vi "Screen_Setup.vi"() -> ()   [LabVIEW 2010]
uses:
  Locked Config.ctl
  030 - EVENTS/EnumFgvEventCommand.ctl
  090 - ERRORS/Ctrls/enumLogAndView.ctl
  <vilib>/Utility/miscctls.llb/LVComboBoxStrsAndValuesArrayTypeDef.ctl
  050 - CONFIG/00 - ApplicationConfig/Ctrls/EnumFgvConfigCommand.ctl
  080 - TOOLS/Traduction/Dictionnary/EnumCommandDictionnaire.ctl
  030 - EVENTS/03 - ToMessageHandlerProcess/enumMessageCriticity.ctl
  030 - EVENTS/03 - ToMessageHandlerProcess/ToMessageHandlerEvent.ctl
  enumScreen.ctl
panel:
  in  "Locked ?":T1
  in  "Répertoire des données":path
  in  "Langue":string(combo)
  in  "Nombre MAX de message par fichier":u16
  in  "Nombre max de fichiers LOG":u16
  in  "Cfg":string
  in  "Bouton menu principal":bool
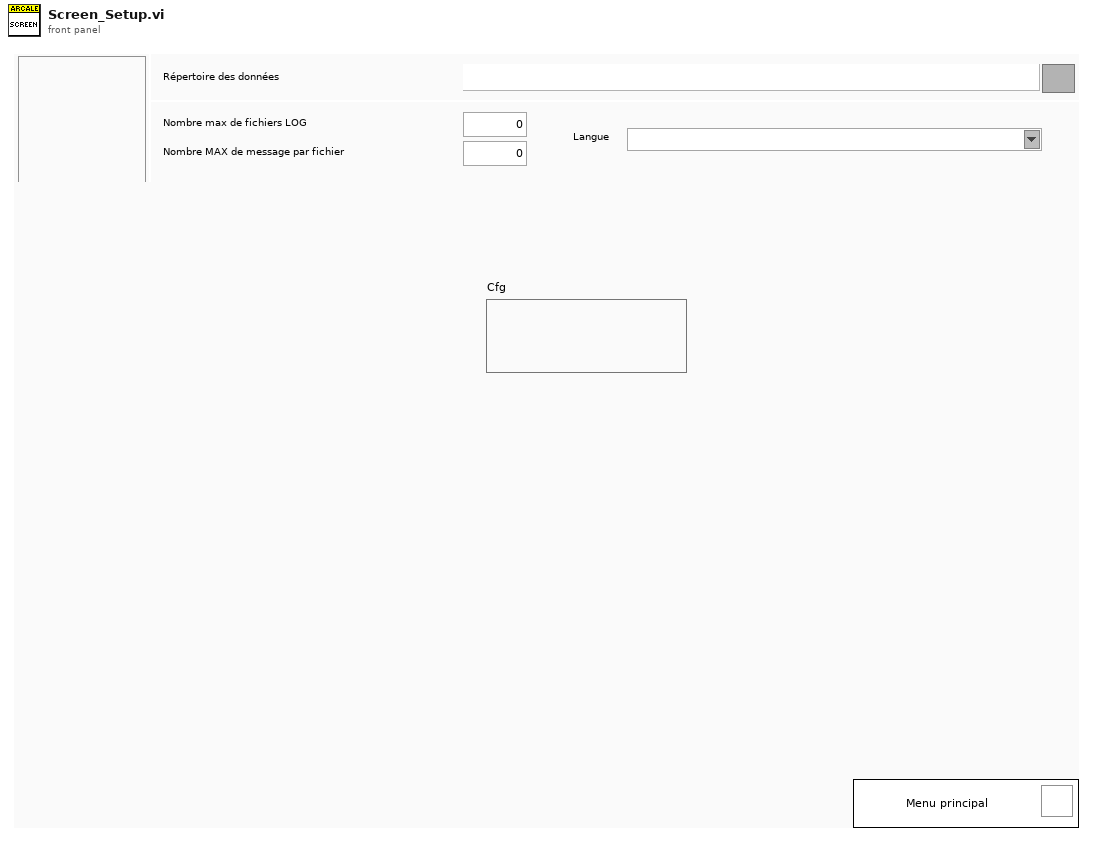
[diagram p1: front panel]
types:
  T1 = typedef "Locked Config.ctl" = bool
  T2 = typedef "enumLogAndView.ctl" = enum16{"Log only", "Log and view"}
  T3 = typedef "EnumFgvEventCommand.ctl" = enum16{"Setup", "Cleanup", "Get"}
  T4 = typedef "LVComboBoxStrsAndValuesArrayTypeDef.ctl" = cluster{"String":string, "Value":string}[]
  T5 = typedef "EnumFgvConfigCommand.ctl" = enum16{"Load", "Get", "Set", "Save To Disk"}
  T6 = typedef "ApplicationConfig.ctl" = cluster{"Data Path":path, "MessageHandlerConfig":T7, "Simulation":bool, "Dictionnary":string}
  T7 = typedef "MessageHandlerConfig.ctl" = cluster{"Max log files":u32, "Max messages per file":u32}
  T8 = typedef "BenchConfig.ctl" = cluster{"Cfg":string}
  T9 = enum8{"Enabled", "Disabled", "Disabled and Grayed Out"}
  T10 = typedef "EnumCommandDictionnaire.ctl" = enum16{"Load", "Translate", "Save", "GetDico", "Set : A traduire = Vrai", "Set : A Traduire = Faux", "SetDico"}
  T11 = typedef "enumMessageCriticity.ctl" = enum16{"No error", "Info", "Warning", "Error", "Fatal error"}
  T12 = typedef "ToMessageHandlerEvent.ctl" = cluster{"date / time":timestamp, "Criticity":T11, "Emitter":string, "Message":string}
  T13 = typedef "enumScreen.ctl" = enum16{"Test screen", "Ecran principal", "LOG", "Setup", "Popup : About", "Popup : View last message", "Popup : WebBrowser help", "Traduction"}
  T14 = typedef "ToScreensCommand.ctl" = enum16{"Stop screen", "Stop all screens"}
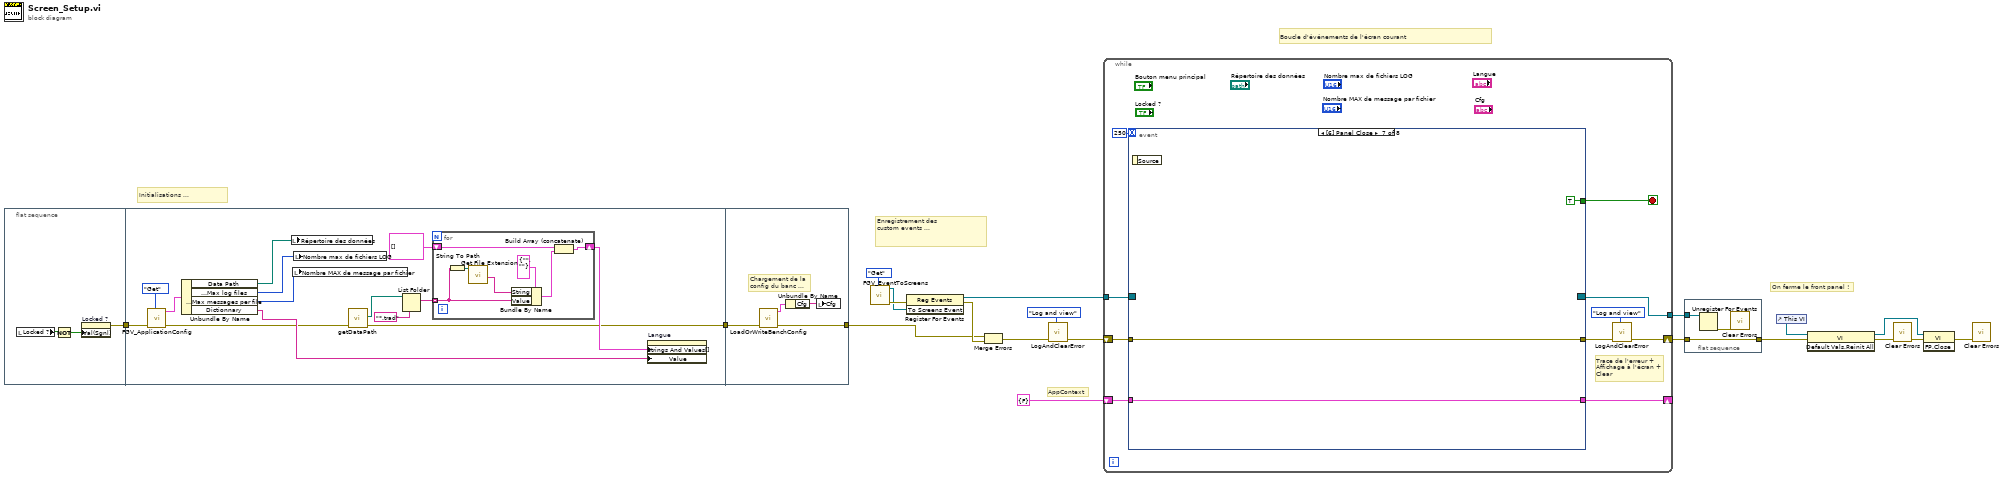
[diagram p0: block diagram]
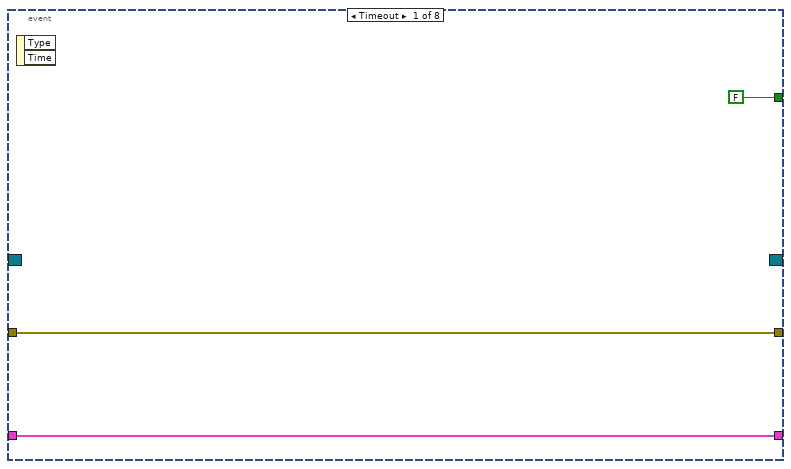
[diagram p2: hidden frame]
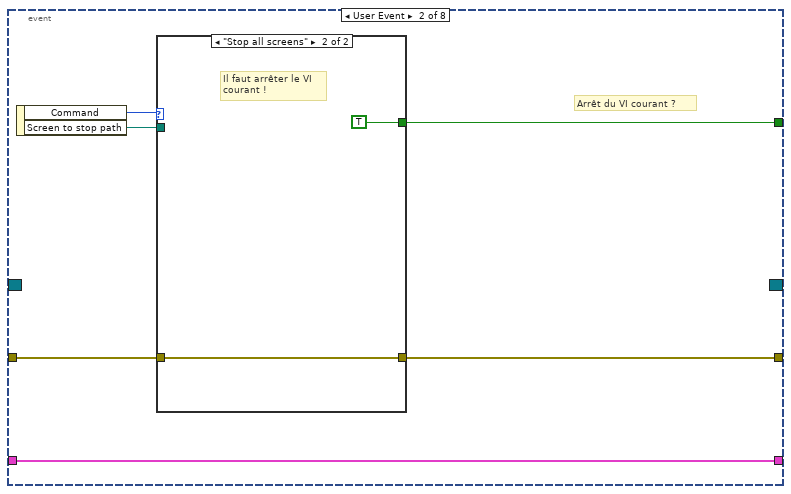
[diagram p3: hidden frame]
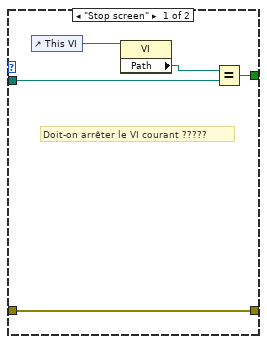
[diagram p4: hidden frame]
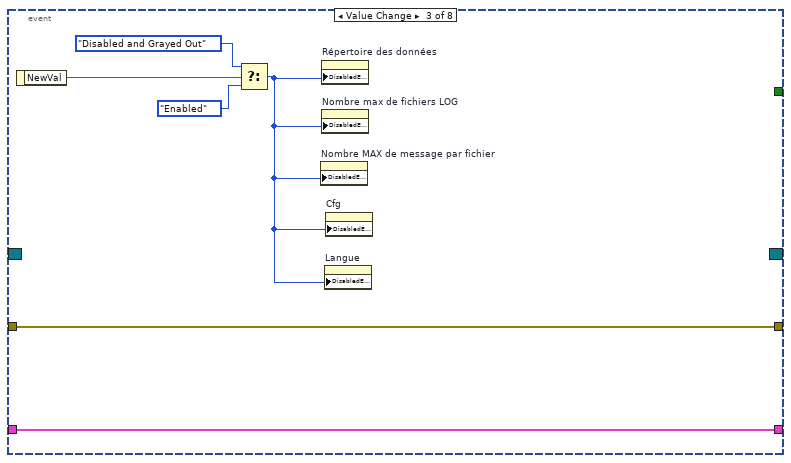
[diagram p5: hidden frame]
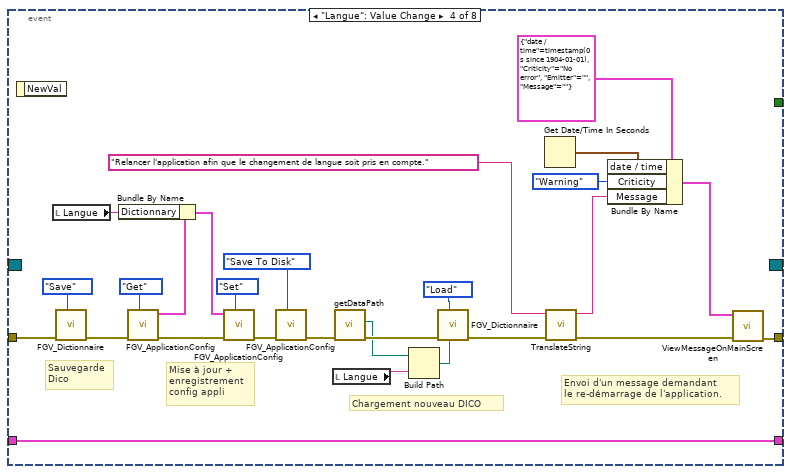
[diagram p6: hidden frame]
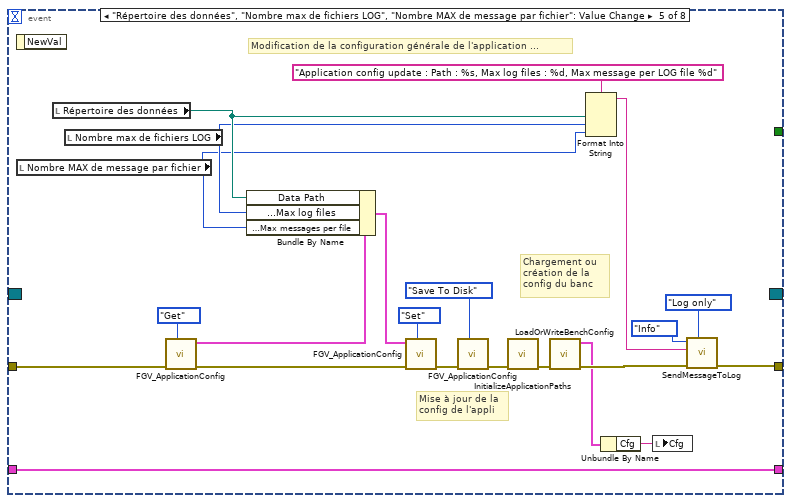
[diagram p7: hidden frame]
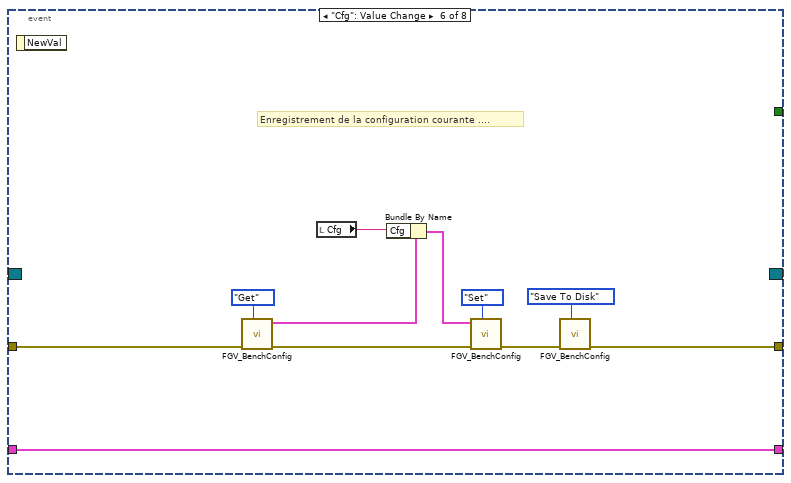
[diagram p8: hidden frame]
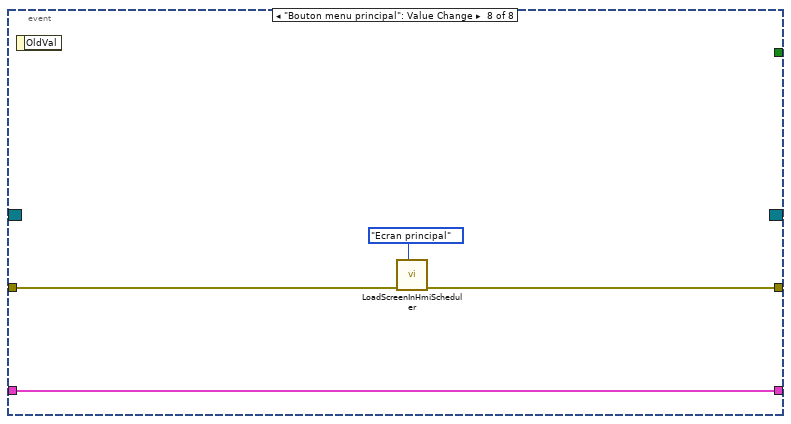
[diagram p9: hidden frame]
diagram:
  # "AppContext"
  # "Enregistrement des\ncustom events ..."
  # "Initialisations ..."
  # "On ferme le front panel !"
  # "Boucle d'événements de l'écran courant"
  n1 = flat-sequence {
    tunnel: [w23] -> w10
    tunnel: w10 -> [w36]
    tunnel: [w25] -> w9
    tunnel: [w47] -> w11
    tunnel: w9 -> [w48]
    frame #0 {
      n2 = local read "Locked ?"() -> (w21:T1)
      n3 = Not(x=w21) -> (.not. x?=w22:T1)
      n4 = property on="Locked ?" class="Bool (strict)"("Val(Sgnl)"=w22) -> (error out=w23:errorcluster)  [unwired: 2 in, 1 out]
    }
    frame #1 {
      n5 = call "FGV_ApplicationConfig.vi"("Command"=EnumFgvConfigCommand."Get", "error in (no error)"=w36) -> ("error out"=w26:errorcluster, "ApplicationConfigOut"=w35:T6)  [unwired: 8 in]
      n6 = Unbundle By Name(w35) -> ("Data Path"=w32:path, "MessageHandlerConfig.Max log files"=w34:u32, "MessageHandlerConfig.Max messages per file"=w33:u32, "Dictionnary"=w30:string)
      n7 = local write "Répertoire des données"(w32) -> ()
      n8 = local write "Nombre MAX de message par fichier"(w33) -> ()
      n9 = local write "Nombre max de fichiers LOG"(w34) -> ()
      n10 = call "getDataPath.vi"("error in (no error)"=w26) -> ("error out"=w25:errorcluster, "DataPath"=w24:path)  [unwired: 9 in]
      n11 = List Folder(path=w24, pattern="*.trad") -> (filenames=w29:string[])  [unwired: 2 in, 3 out]
      n12 = for {
        tunnel: w29 -> [w40] mode=indexing
        shift-right: [w43] -> w27
        shift-left: T4 [] ("Strings And Values []") -> [w44]
        n13 = String To Path(string=w40) -> (path=w39:path)
        n14 = call <vilib>:"Get File Extension.vi"("file"=w39) -> ("filename without extension"=w38:string)  [unwired: 7 in, 3 out]
        n15 = Bundle By Name(cluster=cluster{"String":string, "Value":string} {"String"="", "Value"=""}, "String"=w38, "Value"=w40) -> (w41:cluster{"String":string, "Value":string})
        n16 = Build Array (concatenate)(w44, w41) -> (w43:T4)
      }
      n17 = property on="Langue" class="CmbBox"("Strings And Values[]"=w27, "Value"=w30) -> ()  [unwired: 2 in, 2 out]
    }
    frame #2 {
      # "Chargement de la \nconfig du banc ..."
      n18 = call "LoadOrWriteBenchConfig.vi"("error in (no error)"=w48) -> ("error out"=w47:errorcluster, "BenchConfig"=w46:T8)  [unwired: 9 in]
      n19 = Unbundle By Name(w46) -> ("Cfg"=w45:string)
      n20 = local write "Cfg"(w45) -> ()
    }
  }
  n21 = call "FGV_EventToScreens.vi"("Command"=EnumFgvEventCommand."Get") -> ("error out"=w20:errorcluster, "To Screens Event"=w19:refnum<user-event>)  [unwired: 9 in]
  n22 = register-events(error in=w20, w19) -> (reference out=w18:refnum<event-registration>, error out=w13:errorcluster)  [unwired: 1 in]
  n23 = Merge Errors(w11, w13) -> (w7:errorcluster)
  n24 = call "LogAndClearError.vi"("Log and view ?"=enumLogAndView."Log and view", "error in (no error)"=w7) -> ("error out"=w6:errorcluster)  [unwired: 9 in]
  n25 = while {
    tunnel: w18 -> [w58]
    shift-right: [w52] -> w16
    shift-left: w6 -> [w57]
    tunnel: [w56] -> w17
    shift-right: [w53] -> _
    shift-left: cluster{"Boolean":bool} {"Boolean"=FALSE} ("Cluster") -> [w54]
    stop <- w55 stop-if-true
    # "Trace de l'erreur +\nAffichage à l'écran +\nClear"
    n26 = event shown="[6] Panel Close" {
      selector: w58 -> [_ _ _ _ _ _ _ _]
      dyn-events: [_ _ _ _ _ _ _ _] -> w56
      timeout: 250 -> [_ _ _ _ _ _ _ _]
      tunnel: w57 -> [w61 w66 w77 w90 w127 w139 w142 w147]
      tunnel: [w61 w65 w77 w97 w123 w133 w142 w145] -> w51
      tunnel: [FALSE w63 _ _ _ _ TRUE _] -> w55
      tunnel: w54 -> [w59 w62 w76 w107 w122 w138 w141 w144]
      tunnel: [w59 w62 w76 w107 w122 w138 w141 w144] -> w53
      event Timeout {
        n27 = event-data() -> ()  [unwired: 1 in, 2 out]
      }
      event User Event {
        # "Arrêt du VI courant ?"
        n28 = event-data() -> ("Command"=w67:T14, "Screen to stop path"=w64:path)  [unwired: 1 in]
        n29 = case shown="\"Stop all screens\"" w67 {
          tunnel: w66 -> [w72 w73]
          tunnel: [w72 w73] -> w65
          tunnel: w64 -> [w69 _]
          tunnel: [w68 TRUE] -> w63
          frame "Stop screen" {
            # "Doit-on arrêter le VI courant ?????"
            n30 = control-ref of="This VI"() -> (w71:refnum<vi>)
            n31 = property class="VI"(reference=w71) -> ("Path"=w70:path)  [unwired: 1 in, 2 out]
            n32 = Equal?(x=w70, y=w69) -> (x = y?=w68:bool)
          }
          frame "Stop all screens" {
            # "Il faut arrêter le VI\ncourant !"
          }
        }
      }
      event Value Change {
        n33 = event-data() -> ("NewVal"=w80:T1)  [unwired: 1 in]
        n34 = Select(t=T9."Disabled and Grayed Out" ("Disabled"), s=w80, f=T9."Enabled" ("Disabled")) -> (s? t:f=w75:T9)
        n35 = property on="Nombre MAX de message par fichier" class="DigNum (strict)"("DisabledEnum"=w75) -> ()  [unwired: 2 in, 2 out]
        n36 = property on="Répertoire des données" class="Path"("DisabledEnum"=w75) -> ()  [unwired: 2 in, 2 out]
        n37 = property on="Nombre max de fichiers LOG" class="DigNum (strict)"("DisabledEnum"=w75) -> ()  [unwired: 2 in, 2 out]
        n38 = property on="Langue" class="CmbBox"("DisabledEnum"=w75) -> ()  [unwired: 2 in, 2 out]
        n39 = property on="Cfg" class="Str"("DisabledEnum"=w75) -> ()  [unwired: 2 in, 2 out]
      }
      event "Langue": Value Change {
        # "Envoi d'un message demandant\nle re-démarrage de l'application."
        # "Chargement nouveau DICO"
        # "Mise à jour +\nenregistrement\nconfig appli"
        # "Sauvegarde\nDico"
        n40 = event-data() -> ()  [unwired: 1 in, 1 out]
        n41 = local read "Langue"() -> (w99:string)
        n42 = call "FGV_Dictionnaire.vi"("Command"=EnumCommandDictionnaire."Save", "error in (no error)"=w90) -> ("error out"=w89:errorcluster)  [unwired: 7 in, 2 out]
        n43 = call "FGV_ApplicationConfig.vi"("Command"=EnumFgvConfigCommand."Get", "error in (no error)"=w89) -> ("error out"=w104:errorcluster, "ApplicationConfigOut"=w101:T6)  [unwired: 8 in]
        n44 = Bundle By Name(cluster=w101, "Dictionnary"=w99) -> (w100:T6)
        n45 = call "FGV_ApplicationConfig.vi"("Command"=EnumFgvConfigCommand."Set", "error in (no error)"=w104, "ApplicationConfigIn"=w100) -> ("error out"=w102:errorcluster)  [unwired: 7 in, 1 out]
        n46 = call "FGV_ApplicationConfig.vi"("Command"=EnumFgvConfigCommand."Save To Disk", "error in (no error)"=w102) -> ("error out"=w85:errorcluster)  [unwired: 8 in, 1 out]
        n47 = local read "Langue"() -> (w82:string)
        n48 = call "getDataPath.vi"("error in (no error)"=w85) -> ("error out"=w84:errorcluster, "DataPath"=w83:path)  [unwired: 9 in]
        n49 = Build Path(base path=w83, name or relative path=w82) -> (appended path=w81:path)
        n50 = call "FGV_Dictionnaire.vi"("FichierDictionnaire"=w81, "Command"=EnumCommandDictionnaire."Load", "error in (no error)"=w84) -> ("error out"=w86:errorcluster)  [unwired: 6 in, 2 out]
        n51 = Get Date/Time In Seconds() -> (seconds since 1Jan1904=w94:timestamp)
        n52 = call "TranslateString.vi"("error in (no error)"=w86, "String"="Relancer l'application afin que le changement de langue soit pris en compte.") -> ("error out"=w98:errorcluster, "Translated String"=w92:string)  [unwired: 8 in]
        n53 = Bundle By Name(cluster=T12 {"date / time"=timestamp(0 s since 1904-01-01), "Criticity"=enum."No error", "Emitter"="", "Message"=""} ("Message"), "date / time"=w94, "Criticity"=enumMessageCriticity."Warning", "Message"=w92) -> (w95:T12)
        n54 = call "ViewMessageOnMainScreen.vi"("error in (no error)"=w98, "Message"=w95) -> ("error out"=w97:errorcluster)  [unwired: 9 in]
      }
      event "Répertoire des données", "Nombre max de fichiers LOG", "Nombre MAX de message par fichier": Value Change {
        # "Chargement ou\ncréation de la \nconfig du banc"
        # "Mise à jour de la\nconfig de l'appli"
        # "Modification de la configuration générale de l'application ..."
        n55 = event-data() -> ()  [unwired: 1 in, 1 out]
        n56 = local read "Nombre MAX de message par fichier"() -> (w115:u16)
        n57 = local read "Répertoire des données"() -> (w117:path)
        n58 = local read "Nombre max de fichiers LOG"() -> (w116:u16)
        n59 = call "FGV_ApplicationConfig.vi"("Command"=EnumFgvConfigCommand."Get", "error in (no error)"=w127) -> ("error out"=w126:errorcluster, "ApplicationConfigOut"=w125:T6)  [unwired: 8 in]
        n60 = Bundle By Name(cluster=w125, "Data Path"=w117, "MessageHandlerConfig.Max log files"=w116, "MessageHandlerConfig.Max messages per file"=w115) -> (w124:T6)
        n61 = call "FGV_ApplicationConfig.vi"("Command"=EnumFgvConfigCommand."Set", "error in (no error)"=w126, "ApplicationConfigIn"=w124) -> ("error out"=w111:errorcluster)  [unwired: 7 in, 1 out]
        n62 = call "FGV_ApplicationConfig.vi"("Command"=EnumFgvConfigCommand."Save To Disk", "error in (no error)"=w111) -> ("error out"=w110:errorcluster)  [unwired: 8 in, 1 out]
        n63 = call "InitializeApplicationPaths.vi"("error in (no error)"=w110) -> ("error out"=w114:errorcluster)  [unwired: 10 in]
        n64 = call "LoadOrWriteBenchConfig.vi"("error in (no error)"=w114) -> ("error out"=w113:errorcluster, "BenchConfig"=w108:T8)  [unwired: 9 in]
        n65 = Format Into String(format string="Application config update : Path : %s, Max log files : %d, Max message per LOG file %d", w117, w116, w115) -> (resulting string=w118:string)  [unwired: 2 in, 1 out]
        n66 = Unbundle By Name(w108) -> ("Cfg"=w109:string)
        n67 = local write "Cfg"(w109) -> ()
        n68 = call "SendMessageToLog.vi"("Log and view ?"=enumLogAndView."Log only", "error in (no error)"=w113, "Message"=w118, "Criticity"=enumMessageCriticity."Info") -> ("error out"=w123:errorcluster)  [unwired: 7 in]
      }
      event "Cfg": Value Change {
        # "Enregistrement de la configuration courante ...."
        n69 = event-data() -> ()  [unwired: 1 in, 1 out]
        n70 = call "FGV_BenchConfig.vi"("Command"=EnumFgvConfigCommand."Get", "error in (no error)"=w139) -> ("error out"=w136:errorcluster, "BenchConfigOut"=w132:T8)  [unwired: 8 in]
        n71 = local read "Cfg"() -> (w130:string)
        n72 = Bundle By Name(cluster=w132, "Cfg"=w130) -> (w131:T8)
        n73 = call "FGV_BenchConfig.vi"("Command"=EnumFgvConfigCommand."Set", "error in (no error)"=w136, "BenchConfigIn"=w131) -> ("error out"=w134:errorcluster)  [unwired: 7 in, 1 out]
        n74 = call "FGV_BenchConfig.vi"("Command"=EnumFgvConfigCommand."Save To Disk", "error in (no error)"=w134) -> ("error out"=w133:errorcluster)  [unwired: 8 in, 1 out]
      }
      event Panel Close {
        n75 = event-data() -> ()  [unwired: 1 in, 1 out]
      }
      event "Bouton menu principal": Value Change {
        n76 = event-data() -> ()  [unwired: 1 in, 1 out]
        n77 = call "LoadScreenInHmiScheduler.vi"("Enum Screen"=enumScreen."Ecran principal", "error in (no error)"=w147) -> ("error out"=w145:errorcluster)  [unwired: 9 in]
      }
    }
    n78 = call "LogAndClearError.vi"("Log and view ?"=enumLogAndView."Log and view", "error in (no error)"=w51) -> ("error out"=w52:errorcluster)  [unwired: 9 in]
  }
  n79 = flat-sequence {
    tunnel: w17 -> [w150]
    tunnel: w16 -> [w148]
    tunnel: [w148] -> w3
    frame #0 {
      n80 = Unregister For Events(event registration refnum=w150) -> (error out=w149:errorcluster)  [unwired: 1 in]
      n81 = call <vilib>:"Clear Errors.vi"("error in (no error)"=w149) -> ()  [unwired: 6 in, 1 out]
    }
  }
  n82 = control-ref of="This VI"() -> (w2:refnum<vi>)
  n83 = invoke class="VI" method="Default Vals.Reinit All"(reference=w2, error in=w3) -> (reference out=w1:refnum<vi>, error out=w5:errorcluster)  [unwired: 1 in, 1 out]
  n84 = call <vilib>:"Clear Errors.vi"("error in (no error)"=w5) -> ("error out"=w4:errorcluster)  [unwired: 6 in]
  n85 = invoke class="VI" method="FP.Close"(reference=w1, error in=w4) -> (error out=w15:errorcluster)  [unwired: 1 in, 2 out]
  n86 = call <vilib>:"Clear Errors.vi"("error in (no error)"=w15) -> ()  [unwired: 6 in, 1 out]
